vi "set.vi"(8 "error in (no error)":errorcluster, 10 "user options":T1, 11 "Ring Ref":refnum<vi>[](array[refnum])) -> (0 "error out":errorcluster)   [LabVIEW 2024]
uses:
  controls/ring data.ctl
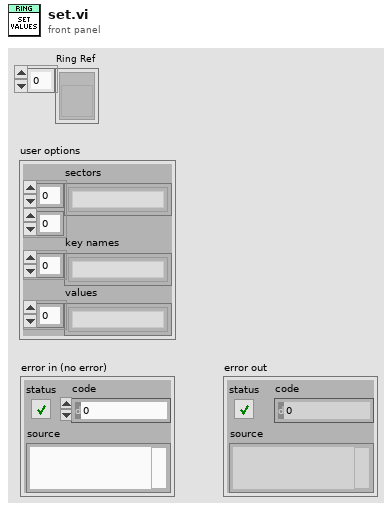
[diagram p1: front panel]
types:
  T1 = typedef "ring data.ctl" = cluster{"sectors":string[][], "key names":string[], "values":string[]}
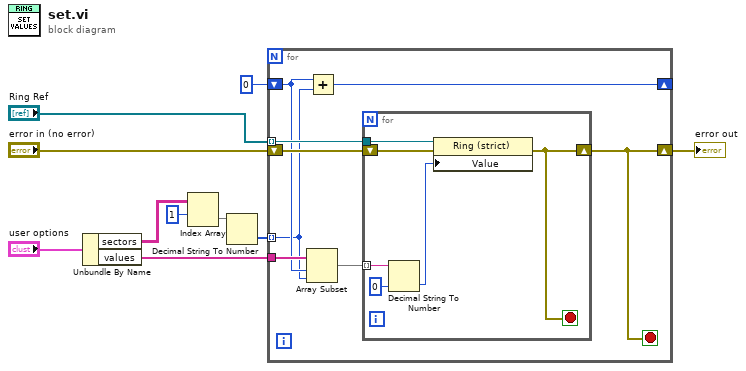
[diagram p0: block diagram]
diagram:
  n1 = Unbundle By Name("user options") -> ("sectors"=w2:string[][], "values"=w1:string[])
  n2 = Index Array(array=w2, index (row)=1) -> (element=w7:string[])  [unwired: 1 in]
  n3 = Decimal String To Number(string=w7) -> (number=w8:i32[])  [unwired: 2 in, 1 out]
  n4 = for {
    tunnel: "Ring Ref" -> [w18] mode=indexing
    shift-right: [w16] -> w10
    shift-left: "error in (no error)" -> [w17]
    tunnel: w8 -> [w12] mode=indexing
    tunnel: w1 -> [w14]
    shift-right: [w15] -> _
    shift-left: 0 -> [w13]
    stop <- w16 stop-if-true
    n5 = Array Subset(array=w14, index=w13, length=w12) -> (w11:string[])
    n6 = Add(x=w13, y=w12) -> (x+y=w15:i32)
    n7 = for {
      tunnel: w18 -> [w24]
      tunnel: w11 -> [w22] mode=indexing
      shift-right: [w19] -> w16
      shift-left: w17 -> [w23]
      stop <- w19 stop-if-true
      n8 = Decimal String To Number(string=w22, default (0L)=u16 0 ("default (0 I32)")) -> (number=w20:u16)  [unwired: 1 in, 1 out]
      n9 = property on="Property Node" class="Ring (strict)"(reference=w24, error in=w23, "Value"=w20) -> (error out=w19:errorcluster)  [unwired: 1 out]
    }
  }
  "error out" <- w10
